vi "file - read-write - list of lines.vi"(7 "read/write control":T1, 9 "header":string, 10 "list of lines IN":string[](array[string]), 11 "file path":path=path "\\\\rus-one\\newdata/data/Ultrasound/Experiment/ProbeTest/Probe10/Hg1201-6-C185-550Cair-3c-83K/sweep3/9w/3366_a.dat") -> (1 "header OUT":string, 2 "list of lines OUT":string[](array[string]))   [LabVIEW 2015]
uses:
  file -- read-write control.ctl
  <vilib>/Utility/file.llb/Read From Spreadsheet File (string).vi
  <vilib>/Utility/file.llb/Write To Spreadsheet File (string).vi
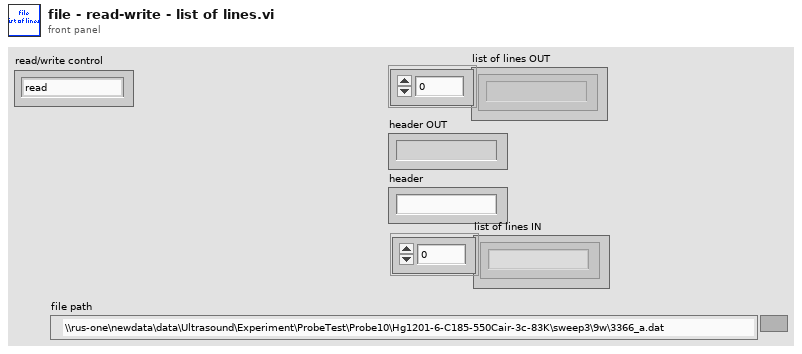
[diagram p1: front panel]
types:
  T1 = typedef "file -- read-write control.ctl" = enum16{"read", "write all", "append one line"}
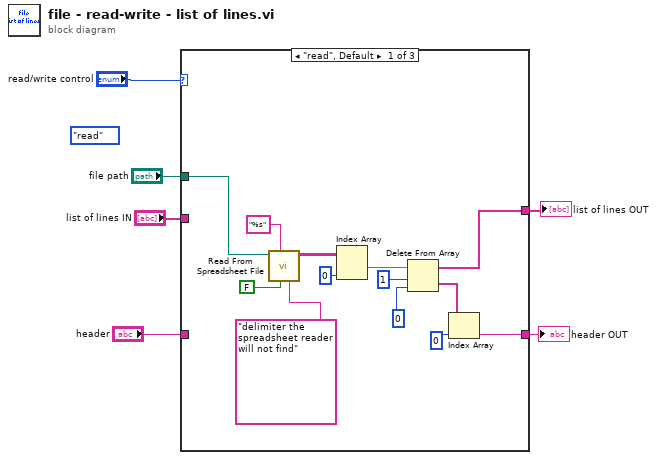
[diagram p0: block diagram]
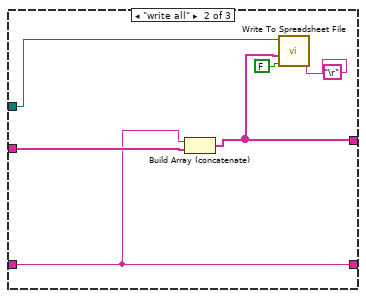
[diagram p2: hidden frame]
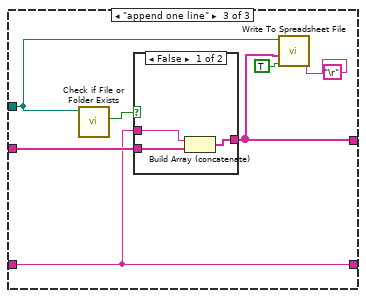
[diagram p3: hidden frame]
diagram:
  (unwired) file_--_read-write_control."read" ("read/write control")
  n1 = case shown="\"read\", Default" "read/write control" {
    tunnel: "file path" -> [w12 w23 w29]
    tunnel: [w8 w21 w27] -> w5
    tunnel: [w7 w20 w26] -> w4
    tunnel: "header" -> [_ w20 w26]
    tunnel: "list of lines IN" -> [_ w22 w28]
    frame "read", Default {
      n2 = call-poly <vilib>:"Read From Spreadsheet File.vi"("delimiter (\\t)"="delimiter the spreadsheet reader will not find" ("delimiter (\\t)"), "transpose (no:F)"=FALSE ("append to file? (new file:F)"), "format (%s)"="%s", "file path (dialog if empty)"=w12) -> ("all rows"=w17:string[][])  [unwired: 3 in, 4 out]
      n3 = Index Array(array=w17, index (col)=0 ("disabled index (col)")) -> (element=w15:string[])  [unwired: 1 in]
      n4 = Delete From Array(array=w15, length=1, index=0) -> (deleted portion=w10:string[], array with subset deleted=w8:string[])
      n5 = Index Array(array=w10, index=0 ("disabled index (col)")) -> (element=w7:string)
    }
    frame "write all" {
      n6 = Build Array (concatenate)(w20, w22) -> (w21:string[])
      n7 = call-poly <vilib>:"Write To Spreadsheet File.vi"("delimiter (\\t)"="\r", "append to file? (new file:F)"=FALSE, "1D data"=w21, "file path (dialog if empty)"=w23) -> ()  [unwired: 4 in, 1 out]
    }
    frame "append one line" {
      n8 = call <vilib>:"Check if File or Folder Exists.vi"("path"=w29) -> ("file or folder exists?"=w30:bool)  [unwired: 8 in, 2 out]
      n9 = case shown="False" w30 {
        tunnel: w28 -> [w35 w36]
        tunnel: w26 -> [w34 _]
        tunnel: [w33 w36] -> w27
        frame False {
          n10 = Build Array (concatenate)(w34, w35) -> (w33:string[])
        }
        frame True {
        }
      }
      n11 = call-poly <vilib>:"Write To Spreadsheet File.vi"("delimiter (\\t)"="\r", "append to file? (new file:F)"=TRUE, "1D data"=w27, "file path (dialog if empty)"=w29) -> ()  [unwired: 4 in, 1 out]
    }
  }
  "list of lines OUT" <- w5
  "header OUT" <- w4
